vi "计算器进阶.vi"() -> ()   [LabVIEW 2018]
panel:
  out "操作临时值":string
  out "输入临时值":string
  out "过程显示":string
  out "结果":string
  out "输入2":string
  out "输入1":string
  in  "等于":bool
  in  "清除":bool
  in  "操作/":bool
  in  "操作*":bool
  in  "操作-":bool
  in  "操作+":bool
  in  "小数点":bool
  in  "数字0":bool
  in  "操作±":bool
  in  "数字 9":bool
  in  "数字 8":bool
  in  "数字7":bool
  in  "数字 6":bool
  in  "数字 5":bool
  in  "数字4":bool
  in  "数字 3":bool
  in  "数字 2":bool
  in  "数字1":bool
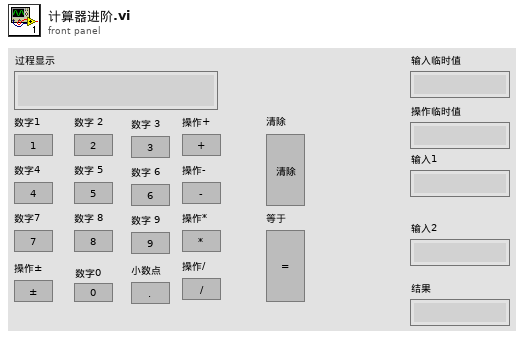
[diagram p1: front panel]
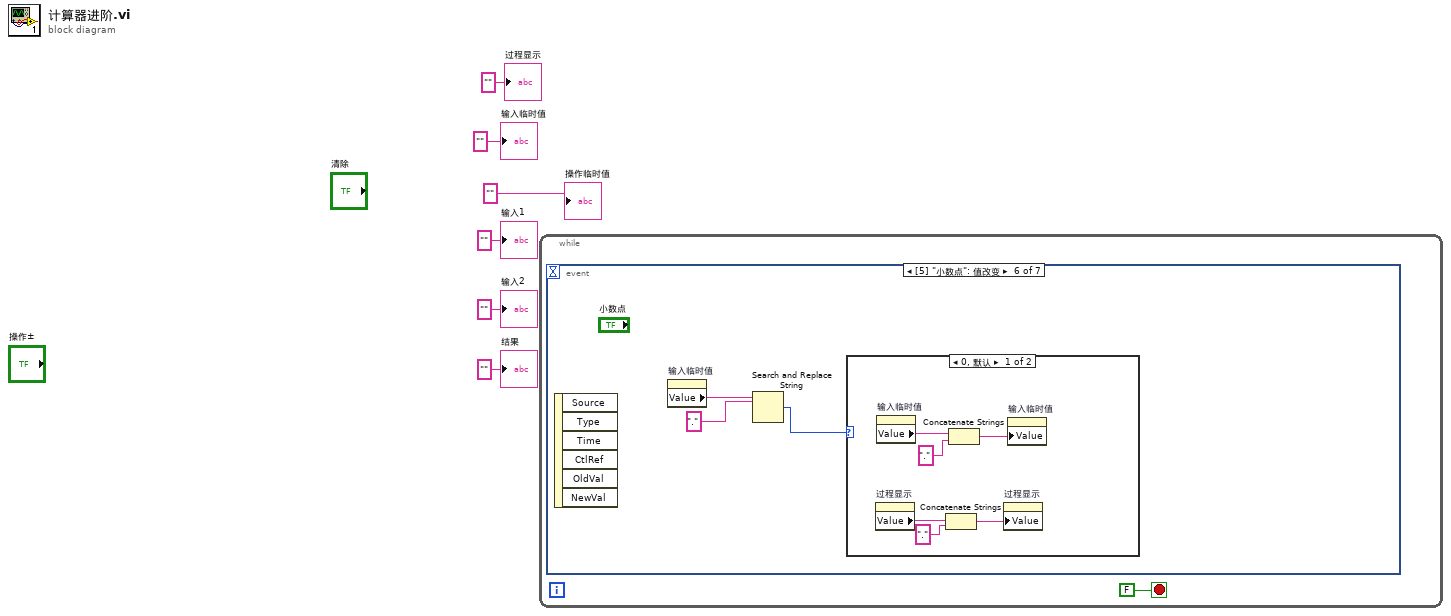
[diagram p0: block diagram]
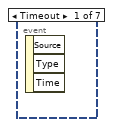
[diagram p2: hidden frame]
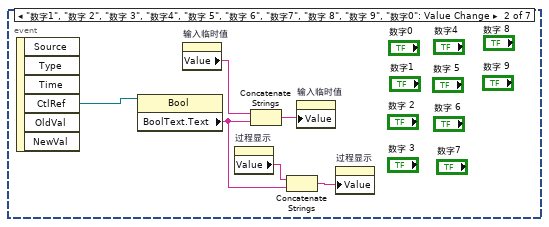
[diagram p3: hidden frame]
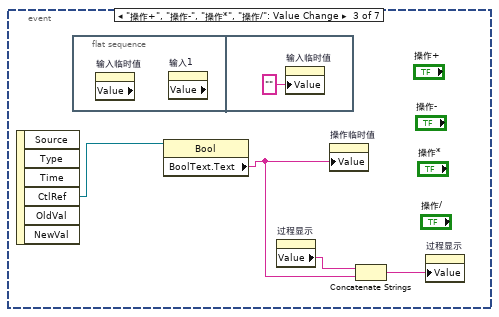
[diagram p4: hidden frame]
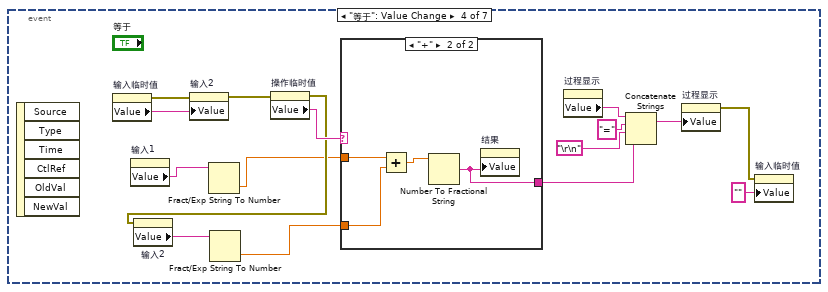
[diagram p5: hidden frame]
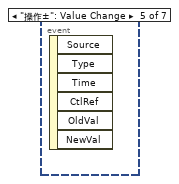
[diagram p7: hidden frame]
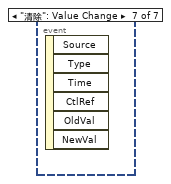
[diagram p9: hidden frame]
diagram:
  n1 = while {
    stop <- FALSE stop-if-true
    n2 = event shown="[5] \"小数点\": 值改变" {
      selector: _ -> [_ _ _ _ _ _ _]
      dyn-events: _ -> [_ _ _ _ _ _ _]
      timeout: _ -> [_ _ _ _ _ _ _]
      event Timeout {
        n3 = event-data() -> ()  [unwired: 1 in, 3 out]
      }
      event "数字1", "数字 2", "数字 3", "数字4", "数字 5", "数字 6", "数字7", "数字 8", "数字 9", "数字0": Value Change {
        n4 = event-data() -> ("CtlRef"=w13:refnum<vi>)  [unwired: 1 in, 5 out]
        n5 = property class="Bool"(reference=w13) -> ("BoolText.Text"=w8:string)  [unwired: 1 in, 2 out]
        n6 = property on="输入临时值" class="Str"() -> ("Value"=w11:string)  [unwired: 2 in, 2 out]
        n7 = property on="过程显示" class="Str"() -> ("Value"=w9:string)  [unwired: 2 in, 2 out]
        n8 = Concatenate Strings(w11, w8) -> (w12:string)
        n9 = Concatenate Strings(w9, w8) -> (w10:string)
        n10 = property on="输入临时值" class="Str"("Value"=w12) -> ()  [unwired: 2 in, 2 out]
        n11 = property on="过程显示" class="Str"("Value"=w10) -> ()  [unwired: 2 in, 2 out]
      }
      event "操作+", "操作-", "操作*", "操作/": Value Change {
        n12 = event-data() -> ("CtlRef"=w17:refnum<vi>)  [unwired: 1 in, 5 out]
        n13 = flat-sequence {
          frame #0 {
            n14 = property on="输入临时值" class="Str" props=["Value"]() -> ()  [unwired: 2 in, 3 out]
            n15 = property on="输入1" class="Str" props=["Value"]() -> ()  [unwired: 2 in, 3 out]
          }
          frame #1 {
            n16 = property on="输入临时值" class="Str"("Value"="" ("输入临时值")) -> ()  [unwired: 2 in, 2 out]
          }
        }
        n17 = property class="Bool"(reference=w17) -> ("BoolText.Text"=w14:string)  [unwired: 1 in, 2 out]
        n18 = property on="过程显示" class="Str"() -> ("Value"=w16:string)  [unwired: 2 in, 2 out]
        n19 = property on="操作临时值" class="Str"("Value"=w14) -> ()  [unwired: 2 in, 2 out]
        n20 = Concatenate Strings(w16, w14) -> (w15:string)
        n21 = property on="过程显示" class="Str"("Value"=w15) -> ()  [unwired: 2 in, 2 out]
      }
      event "等于": Value Change {
        n22 = event-data() -> ()  [unwired: 1 in, 6 out]
        n23 = property on="输入临时值" class="Str"() -> (error out=w26:errorcluster, "Value"=w34:string)  [unwired: 2 in, 1 out]
        n24 = property on="输入1" class="Str"() -> ("Value"=w32:string)  [unwired: 2 in, 2 out]
        n25 = property on="输入2" class="Str"(error in=w26, "Value"=w34) -> (error out=w30:errorcluster)  [unwired: 1 in, 1 out]
        n26 = Fract/Exp String To Number(string=w32) -> (number=w28:dbl)  [unwired: 3 in, 1 out]
        n27 = property on="操作临时值" class="Str"(error in=w30) -> (error out=w29:errorcluster, "Value"=w33:string)  [unwired: 1 in, 1 out]
        n28 = property on="输入2" class="Str"(error in=w29) -> ("Value"=w31:string)  [unwired: 1 in, 2 out]
        n29 = Fract/Exp String To Number(string=w31) -> (number=w27:dbl)  [unwired: 3 in, 1 out]
        n30 = case shown="\"+\"" w33 {
          tunnel: w28 -> [_ w38]
          tunnel: w27 -> [_ w37]
          tunnel: [_ w35] -> w21
          frame "假", Default {
          }
          frame "+" {
            n31 = Add(x=w38, y=w37) -> (x+y=w36:dbl)
            n32 = Number To Fractional String(number=w36) -> (F-format string=w35:string)  [unwired: 3 in]
            n33 = property on="结果" class="Str"("Value"=w35) -> ()  [unwired: 2 in, 2 out]
          }
        }
        n34 = property on="过程显示" class="Str"() -> ("Value"=w25:string)  [unwired: 2 in, 2 out]
        n35 = Concatenate Strings(w25, "=" ("字符串"), "\r\n", w21) -> (w24:string)
        n36 = property on="过程显示" class="Str"("Value"=w24) -> (error out=w19:errorcluster)  [unwired: 2 in, 1 out]
        n37 = property on="输入临时值" class="Str"(error in=w19, "Value"="" ("输入临时值")) -> ()  [unwired: 1 in, 2 out]
      }
      event "操作±": Value Change {
        n38 = event-data() -> ()  [unwired: 1 in, 6 out]
      }
      event "小数点": Value Change {
        n39 = event-data() -> ()  [unwired: 1 in, 6 out]
        n40 = property on="输入临时值" class="Str"() -> ("Value"=w41:string)  [unwired: 2 in, 2 out]
        n41 = Search and Replace String(input string=w41, search string="." ("搜索字符串")) -> (number of replacements=w39:i32)  [unwired: 6 in, 3 out]
        n42 = case shown="0, 默认" w39 {
          frame 0, Default {
            n43 = property on="过程显示" class="Str"() -> ("Value"=w44:string)  [unwired: 2 in, 2 out]
            n44 = property on="输入临时值" class="Str"() -> ("Value"=w47:string)  [unwired: 2 in, 2 out]
            n45 = Concatenate Strings(w44, "." ("连接的字符串")) -> (w42:string)
            n46 = Concatenate Strings(w47, "." ("连接的字符串")) -> (w45:string)
            n47 = property on="过程显示" class="Str"("Value"=w42) -> ()  [unwired: 2 in, 2 out]
            n48 = property on="输入临时值" class="Str"("Value"=w45) -> ()  [unwired: 2 in, 2 out]
          }
          frame 1 {
          }
        }
      }
      event "清除": Value Change {
        n49 = event-data() -> ()  [unwired: 1 in, 6 out]
      }
    }
  }
  "输入1" <- "" ("输入1")
  "输入2" <- "" ("输入2")
  "结果" <- "" ("结果")
  "过程显示" <- "" ("过程显示")
  "输入临时值" <- "" ("输入临时值")
  "操作临时值" <- "" ("操作临时值")
